vi "Parse In String.vi"(8 "error in (no error)":errorcluster, 11 "Partial JSON (starting with quote)":string) -> (0 "error out":errorcluster, 2 "Rest of JSON":string, 3 "String (incl quotes)":string)   [LabVIEW 2011, in "JSON Value.lvclass"]
doc: "Parse out a JSON String (properly escaped) from the front of the incoming JSON fragment (must have a quote as first char)."
uses:
  JSON Value/JSON Value.lvclass
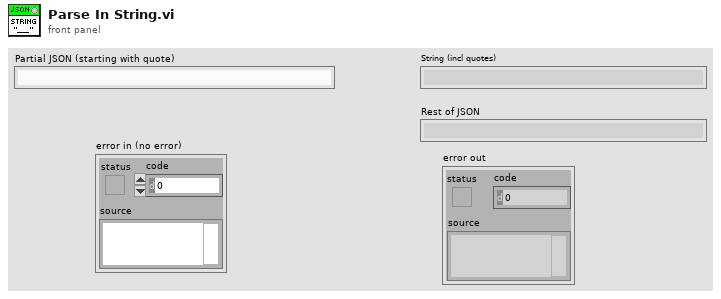
[diagram p1: front panel]
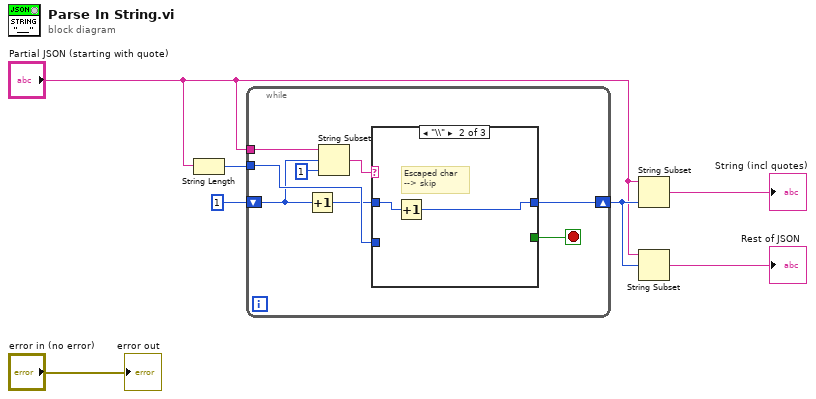
[diagram p0: block diagram]
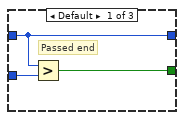
[diagram p2: hidden frame]
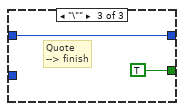
[diagram p3: hidden frame]
diagram:
  n1 = String Length(string="Partial JSON (starting with quote)") -> (length=w3:i32)
  n2 = while {
    tunnel: "Partial JSON (starting with quote)" -> [w15]
    shift-right: [w12] -> w6
    shift-left: 1 -> [w8]
    tunnel: w3 -> [w11]
    stop <- w10 stop-if-true
    n3 = Increment(x=w8) -> (x+1=w9:i32)
    n4 = String Subset(string=w15, offset (0)=w8, length (rest)=1 ("length (rest)")) -> (substring=w13:string)
    n5 = case shown="\"\\\\\"" w13 {
      tunnel: w9 -> [w18 w20 w22]
      tunnel: [w18 w19 w22] -> w12
      tunnel: w11 -> [w17 _ _]
      tunnel: [w16 _ TRUE] -> w10
      frame Default {
        # "Passed end"
        n6 = Greater?(x=w18, y=w17) -> (0:w16:bool)
      }
      frame "\\" {
        # "Escaped char\n--> skip"
        n7 = Increment(x=w20) -> (x+1=w19:i32)
      }
      frame "\"" {
        # "Quote\n--> finish"
      }
    }
  }
  n8 = String Subset(string="Partial JSON (starting with quote)", length (rest)=w6) -> (substring=→"String (incl quotes)":string)  [unwired: 1 in]
  n9 = String Subset(string="Partial JSON (starting with quote)", offset (0)=w6) -> (substring=→"Rest of JSON":string)  [unwired: 1 in]
  "error out" <- "error in (no error)"
